vi "Read LimitCurrent.vi"(8 "error in (no error)":errorcluster, 11 "PS Driver in":refnum<class "PS Driver.lvclass">) -> (0 "error out":errorcluster, 2 "LimitCurrent":dbl, 3 "PS Driver out":refnum<class "PS Driver.lvclass">)   [LabVIEW 2024, in "PS Driver.lvlib" / "PS Driver.lvclass"]
uses:
  PS Driver.lvclass
  PS Driver.lvclass/PS Driver.ctl
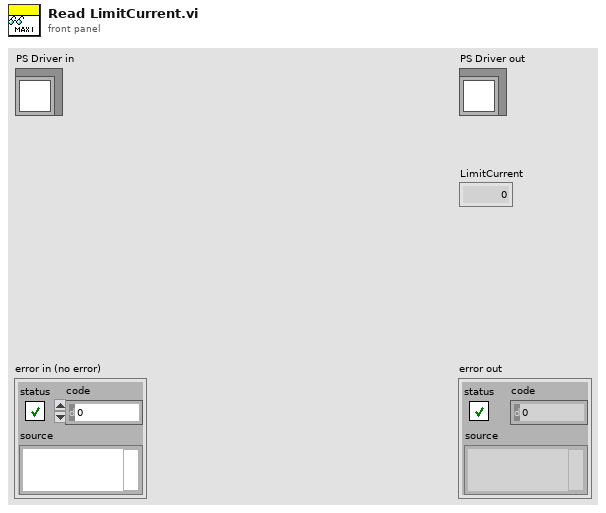
[diagram p1: front panel]
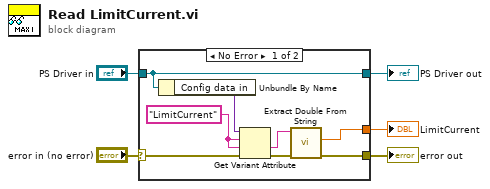
[diagram p0: block diagram]
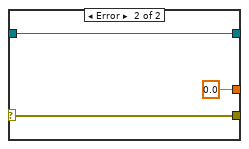
[diagram p2: hidden frame]
diagram:
  n1 = case shown="No Error" "error in (no error)" {
    selector: "error in (no error)" -> [w11 w15]
    tunnel: [w6 w15] -> w4
    tunnel: [w13 w16] -> w2
    tunnel: "PS Driver in" -> [w13 w16]
    tunnel: [w8 0.0] -> w1
    frame No Error {
      w10 = "LimitCurrent" ("name")
      n2 = Unbundle By Name(w13) -> ("Config data in"=w12:variant)
      n3 = Get Variant Attribute(Variant=w12, name=w10, default value (empty Variant)=w10, error in=w11) -> (value=w9:string, error out=w7:errorcluster)  [unwired: 2 out]
      n4 = call "Extract Double From String.vi"("error in"=w7, "string"=w9) -> ("error out"=w6:errorcluster, "floating pt. number"=w8:dbl)  [unwired: 2 in, 2 out]
    }
    frame Error {
    }
  }
  "error out" <- w4
  "PS Driver out" <- w2
  "LimitCurrent" <- w1
